vi "Read-2XY Data.vi"(8 "read config":T2(array[cluster]), 11 "appended path":path) -> (0 "当前XY":cluster{"X":dbl, "Y":dbl, "Z":dbl}[](array[cluster]), 3 "点位":T1)   [LabVIEW 2011]
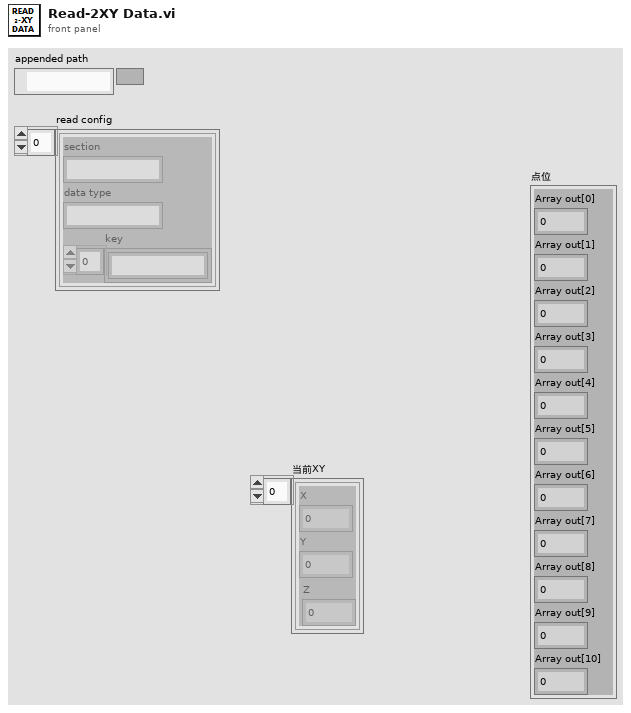
[diagram p1: front panel]
types:
  T1 = cluster{"Array out[0]":dbl, "Array out[1]":dbl, "Array out[2]":dbl, "Array out[3]":dbl, "Array out[4]":dbl, "Array out[5]":dbl, "Array out[6]":dbl, "Array out[7]":dbl, "Array out[8]":dbl, "Array out[9]":dbl, "Array out[10]":dbl}
  T2 = cluster{"section":string, "data type":string, "key":string[]}[]
  T3 = cluster{"Boolean":bool[], "Double":dbl[], "I32":i32[], "Path":path[], "String":string[], "U32":u32[]}[]
  T4 = cluster{"Boolean":bool[], "Double":dbl[], "I32":i32[], "Path":path[], "String":string[], "U32":u32[]}
  T5 = cluster{"Array out[0]":string, "Array out[1]":string, "Array out[2]":string, "Array out[3]":string, "Array out[4]":string, "Array out[5]":string, "Array out[6]":string, "Array out[7]":string, "Array out[8]":string, "Array out[9]":string, "Array out[10]":string}
  T6 = cluster{"String in":string, "String in":string, string}
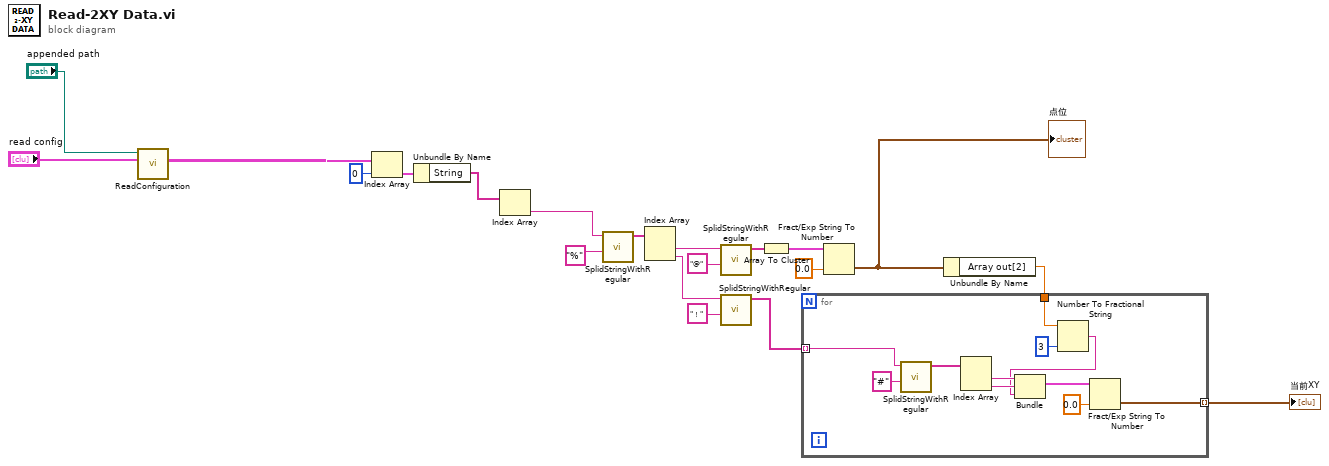
[diagram p0: block diagram]
diagram:
  n1 = call "ReadConfiguration.vi"("read config"="read config", "configuration file path"="appended path") -> ("data out"=w6:T3)  [unwired: 2 in, 3 out]
  n2 = Index Array(array=w6, index=0 ("索引")) -> (element=w5:T4)
  n3 = Unbundle By Name(w5) -> ("String"=w12:string[])
  n4 = Index Array(array=w12) -> (element=w11:string)  [unwired: 1 in]
  n5 = call "SplidStringWithRegular.vi"("regular expression"="%", "String in"=w11) -> ("Array out"=w10:string[])  [unwired: 9 in]
  n6 = Index Array(array=w10) -> (element #1=w14:string, element #2=w18:string)  [unwired: 2 in]
  n7 = call "SplidStringWithRegular.vi"("regular expression"="@", "String in"=w14) -> ("Array out"=w15:string[])  [unwired: 9 in]
  n8 = call "SplidStringWithRegular.vi"("regular expression"="！", "String in"=w18) -> ("Array out"=w20:string[])  [unwired: 9 in]
  n9 = Array To Cluster(array=w15) -> (cluster=w16:T5)
  n10 = Fract/Exp String To Number(string=w16, default (0 dbl)=0.0 ("默认(0 DBL)")) -> (number=w3:T1)  [unwired: 2 in, 1 out]
  "点位" <- w3
  n11 = Unbundle By Name(w3) -> ("Array out[2]"=w2:dbl)
  n12 = for {
    tunnel: w20 -> [w30] mode=indexing
    tunnel: [w24] -> w1 mode=indexing
    tunnel: w2 -> [w23]
    n13 = call "SplidStringWithRegular.vi"("regular expression"="#", "String in"=w30) -> ("Array out"=w29:string[])  [unwired: 9 in]
    n14 = Index Array(array=w29) -> (element #1=w27:string, element #2=w28:string)  [unwired: 2 in]
    n15 = Number To Fractional String(number=w23, precision (6)=i16 3 ("精度(6)")) -> (F-format string=w21:string)  [unwired: 2 in]
    n16 = Bundle("String in"=w27, "String in"=w28, w21) -> (w26:T6)  [unwired: 1 in]
    n17 = Fract/Exp String To Number(string=w26, default (0 dbl)=0.0 ("默认(0 DBL)")) -> (number=w24:cluster{"String in":dbl, "String in":dbl, dbl})  [unwired: 2 in, 1 out]
  }
  "当前XY" <- w1
